vi "Nominal Value Write Array.vi"(0 "Voltage Nominal Value in":refnum<class "Voltage Nominal Value.lvclass">, 1 "Voltage Nominal Value Value":dbl[](array[numeric]), 3 "error in":errorcluster) -> (7 "Voltage Nominal Value out":refnum<class "Voltage Nominal Value.lvclass">, 10 "error out":errorcluster)   [LabVIEW 2023, in "Voltage Nominal Value.lvclass"]
uses:
  Voltage Nominal Value.lvclass
  Parents/Nominal Value/Nominal Value.lvclass
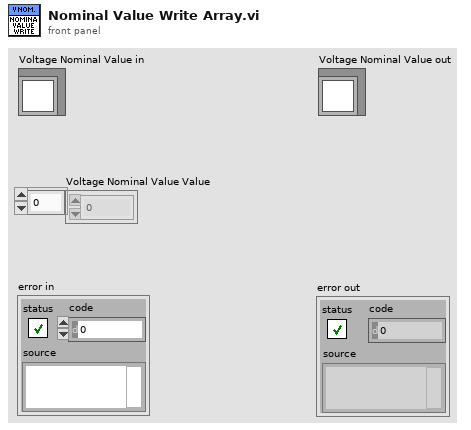
[diagram p1: front panel]
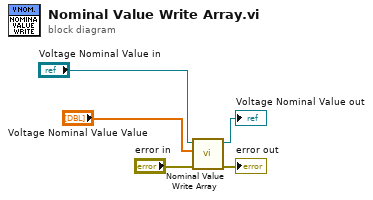
[diagram p0: block diagram]
diagram:
  n1 = call-parent "Nominal Value Write Array.vi"("Nominal Value in"="Voltage Nominal Value in", "Nominal Value Value"="Voltage Nominal Value Value", "error in"="error in") -> ("Nominal Value out"=→"Voltage Nominal Value out":refnum<class "Voltage Nominal Value.lvclass">, "error out"=→"error out":errorcluster)  [unwired: 6 in]
